vi "JogForMinimum.vi"(0 "TLCamera reference in":refnum<k24>, 1 "MotorController in":refnum<class "MotorController.lvclass">, 5 "Axis":T1, 7 "Exposure (us)":u32, 11 "Error In":errorcluster) -> (3 "MotorController Out":refnum<class "MotorController.lvclass">, 4 "TLCamera reference out":refnum<k24>, 6 "Jog Steps":i32[](array[numeric]), 8 "Amplitudes":dbl[](array[numeric]), 10 "Jog of Minimum":i32, 15 "Error Out":errorcluster)   [LabVIEW 2019]
uses:
  MotorController.lvclass
  Axes_enum_typedef.ctl
  C:/Users/jleeman/git_repos/CAxis_Machine/C-Axis LabView Controller/Library_X64/Thorlabs.TSI.TLCameraInterfaces.dll
  Library_X64/Thorlabs.TSI.TLCameraInterfaces.dll
panel:
  out "current jog cumulative":i32
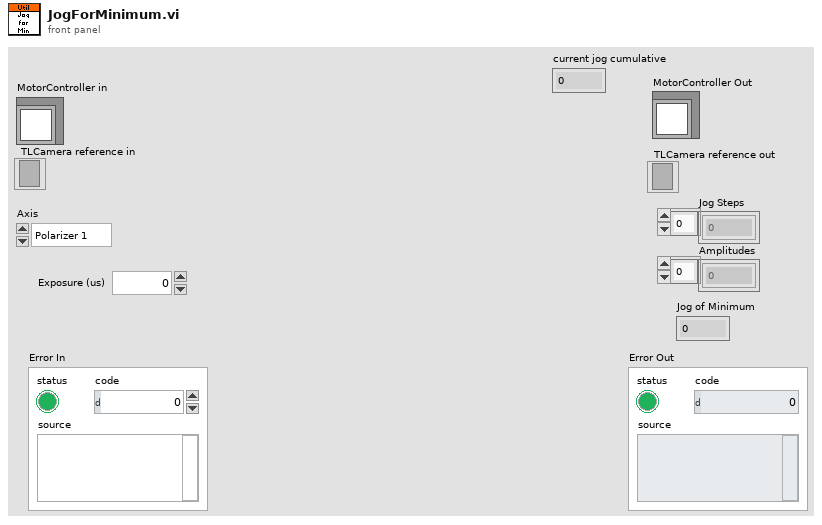
[diagram p1: front panel]
types:
  T1 = typedef "Axes_enum_typedef.ctl" = enum16{"Polarizer 1", "Polarizer 2", "Sample", "Stage"}
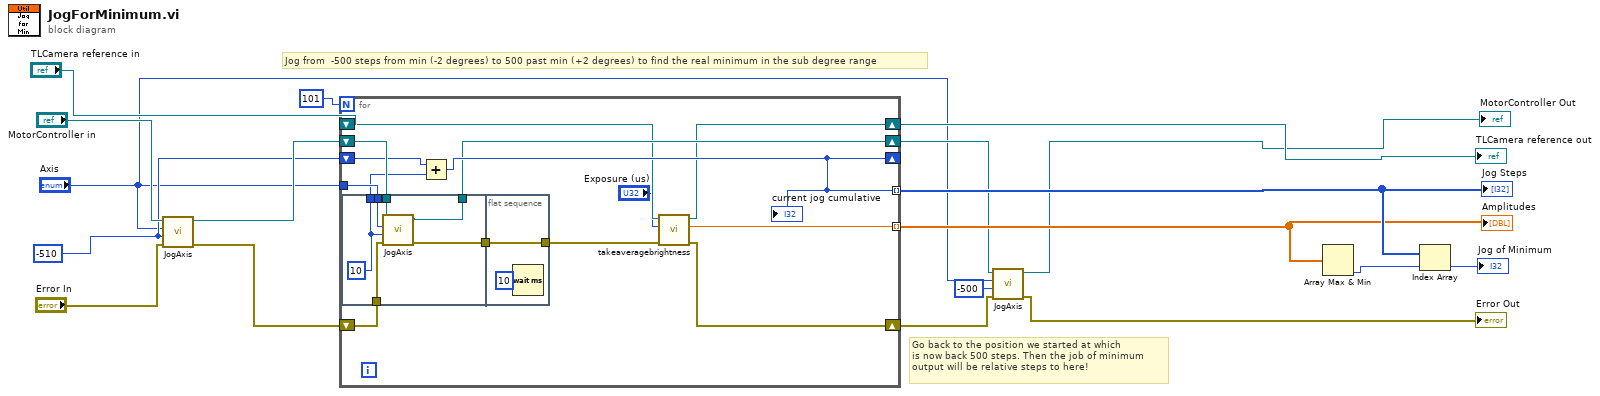
[diagram p0: block diagram]
diagram:
  w7 = -510 ("Steps")
  # "Go back to the position we started at which \nis now back 500 steps. Then the job of minimum\noutput will be relative steps to here!"
  # "Jog from  -500 steps from min (-2 degrees) to 500 past min (+2 degrees) to find the real minimum in the sub degree range"
  n1 = call "JogAxis.vi"("error in (no error)"="Error In", "Steps"=w7, "Axis"="Axis", "MotorController in"="MotorController in") -> ("error out"=w9:errorcluster, "MotorController out"=w10:refnum<class "MotorController.lvclass">)  [unwired: 6 in]
  n2 = for {
    N: 101 -> [_]
    tunnel: "Axis" -> [w31]
    shift-right: [w28] -> _
    shift-left: w7 -> [w30]
    shift-right: [w24] -> w13
    shift-left: "TLCamera reference in" -> [w25]
    tunnel: [w28] -> w12 mode=indexing
    shift-right: [w26] -> w4
    shift-left: w10 -> [w32]
    shift-right: [w22] -> w6
    shift-left: w9 -> [w27]
    tunnel: [w23] -> w8 mode=indexing
    n3 = flat-sequence {
      tunnel: w32 -> [w38]
      tunnel: w31 -> [w37]
      tunnel: [w36] -> w29
      tunnel: w27 -> [w35]
      tunnel: [w34] -> w26
      tunnel: [w33] -> w19
      tunnel: [w40] -> w21
      tunnel: w19 -> [w40]
      frame #0 {
        w36 = 10 ("Steps")
        n4 = call "JogAxis.vi"("error in (no error)"=w35, "Steps"=w36, "Axis"=w37, "MotorController in"=w38) -> ("error out"=w33:errorcluster, "MotorController out"=w34:refnum<class "MotorController.lvclass">)  [unwired: 6 in]
      }
      frame #1 {
        n5 = Wait (ms)(milliseconds to wait=u32 10) -> ()  [unwired: 1 out]
      }
    }
    n6 = Add(x=w30, y=w29) -> (x+y=w28:i32)
    "current jog cumulative" <- w28
    n7 = call "takeaveragebrightness.vi"("Error In"=w21, "Exposure (us)"="Exposure (us)", "TLCamera reference in"=w25) -> ("Error Out"=w22:errorcluster, "brightness"=w23:dbl, "TLCamera reference out"=w24:refnum<k24>)  [unwired: 6 in]
  }
  "Jog Steps" <- w12
  "TLCamera reference out" <- w13
  "Amplitudes" <- w8
  n8 = call "JogAxis.vi"("error in (no error)"=w6, "Steps"=-500, "Axis"="Axis", "MotorController in"=w4) -> ("error out"=→"Error Out":errorcluster, "MotorController out"=→"MotorController Out":refnum<class "MotorController.lvclass">)  [unwired: 6 in]
  n9 = Array Max & Min(array=w8) -> (min index (indices)=w14:i32)  [unwired: 3 out]
  n10 = Index Array(array=w12, index=w14) -> (element=→"Jog of Minimum":i32)
